vi "308L-Labview project 1.vi"() -> ()   [LabVIEW 2010]
uses:
  <vilib>/Utility/file.llb/Write To Spreadsheet File (DBL).vi
  <vilib>/Analysis/NI_AALBase.lvlib
panel:
  in  "Save?":bool
  in  "intervals":i32=10
  out "XY Graph":T1(graph)
  in  "Expected random number":dbl
  out "Waveform Graph":dbl[](graph)
  in  "Number of Random Numbers":i32
  out "number (0 to 1) 2":dbl
  out "Number of iterations":i32
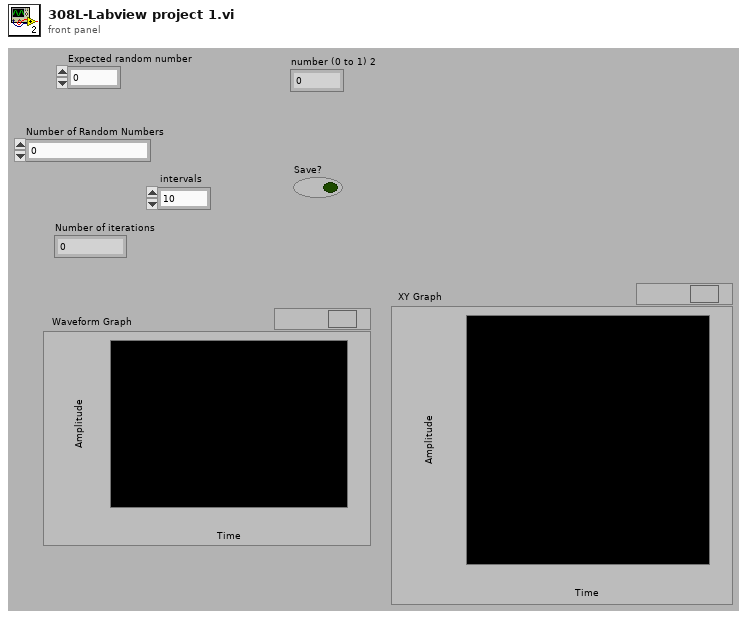
[diagram p1: front panel]
types:
  T1 = cluster{"X Values":dbl[], "Histogram: h(x)":i32[]}
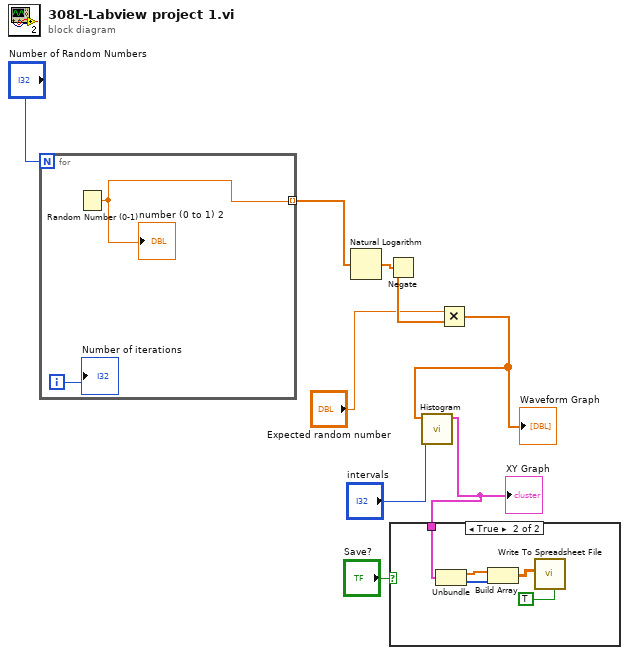
[diagram p0: block diagram]
diagram:
  n1 = for {
    N: "Number of Random Numbers" -> [_]
    tunnel: [w10] -> w8 mode=indexing
    i -> [w11]
    n2 = Random Number (0-1)() -> (number: 0 to 1=w10:dbl)
    "number (0 to 1) 2" <- w10
    "Number of iterations" <- w11
  }
  n3 = Natural Logarithm(1:w8) -> (0:w7:dbl[])
  n4 = Negate(x=w7) -> (-x=w6:dbl[])
  n5 = Multiply(x="Expected random number", y=w6) -> (x*y=w4:dbl[])
  "Waveform Graph" <- w4
  n6 = call <vilib>:"Histogram.vi"("intervals"="intervals", "X"=w4) -> ("Histogram Graph"=w2:T1)  [unwired: 6 in, 3 out]
  "XY Graph" <- w2
  n7 = case shown="True" "Save?" {
    tunnel: w2 -> [_ w16]
    frame False {
    }
    frame True {
      n8 = Unbundle(w16) -> ("X Values"=w15:dbl[], "Histogram: h(x)"=w14:i32[])
      n9 = Build Array(w15, w14) -> (w13:dbl[][])
      n10 = call-poly <vilib>:"Write To Spreadsheet File.vi"("transpose? (no:F)"=TRUE, "2D data"=w13) -> ()  [unwired: 6 in, 1 out]
    }
  }
